vi "Get channel info.vi"(8 "error in":errorcluster) -> (0 "error out":errorcluster, 1 "Cancelled":bool, 3 "Sampling info":T1 {"Channels"."Hi cutoff" items=["500"=500.0, "1k"=1000.0, "5k"=5000.0, "10k"=10000.0, "20k"=20000.0]; "Channels"."Lo cutoff" items=["0.1"=0.1, "1"=1.0, "10"=10.0, "100"=100.0, "300"=300.0]; "Channels"."Gain" items=["x100"=100, "x1000"=1000, "x10000"=10000]})   [LabVIEW 2012]
uses:
  Channel.ctl
  Sampling info.ctl
panel:
  in  "Vel gain in":dbl=0.5 caption="Speed gain"
  in  "Pos gain in":dbl=1.0 caption="Position gain"
  in  "Max accel in":dbl[unit]=17453.292519943294 caption="Maximum acceleration"
  in  "Max speed in":dbl[unit]=87.26646259971648 caption="Maximum speed"
  in  "Steps bit in":u8 caption="Step bit"
  in  "Output frequency in":dbl[unit]=10000.0 caption="Output frequency"
  in  "Counts per rev in":i32=2048 caption="Encoder counts per revolution"
  in  "Motor driver in":string(combo)="US Digital MD2S" caption="Motor driver"
  in  "Steps per rev in":i32=6400 caption="Steps per revolution"
  in  "Cancel":bool
  in  "OK":bool
  in  "Amplifier in":string(combo)="A-M Systems 1700" caption="Amplifier"
  in  "Update frequency in":dbl[unit]=20.0 caption="Update frequency"
  in  "Sampling frequency in":dbl[unit]=5000.0 caption="Sampling frequency"
  in  "Channels in":T2[](array[typedef]) caption="Channels" {"Hi cutoff" items=["500"=500.0, "1k"=1000.0, "5k"=5000.0, "10k"=10000.0, "20k"=20000.0]; "Lo cutoff" items=["0.1"=0.1, "1"=1.0, "10"=10.0, "100"=100.0, "300"=300.0]; "Gain" items=["x100"=100, "x1000"=1000, "x10000"=10000]}
  # "Recording"
  # "Motor"
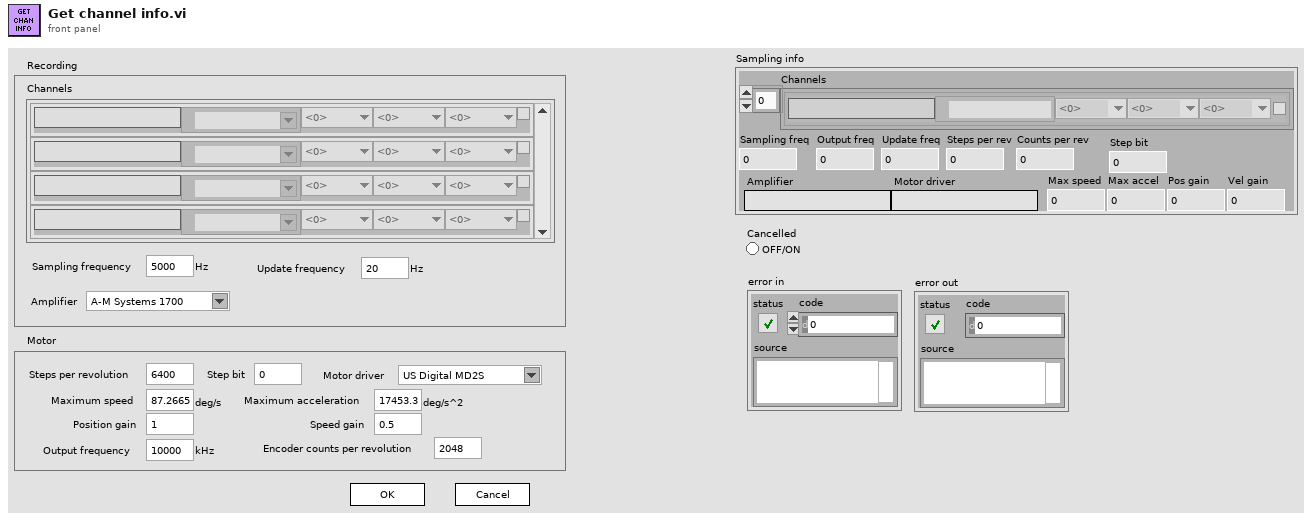
[diagram p1: front panel]
types:
  T1 = typedef "Sampling info.ctl" = cluster{"Channels":T2[], "Sampling freq":i32, "Output freq":i32, "Update freq":i32, "Steps per rev":i32, "Counts per rev":i32, "Amplifier":string, "Motor driver":string, "Step bit":u8, "Max speed":dbl, "Max accel":dbl, "Pos gain":dbl, "Vel gain":dbl}
  T2 = typedef "Channel.ctl" = cluster{"Name":string, "Chan":tag, "Gain":u16, "Lo cutoff":dbl, "Hi cutoff":dbl, "Notch":bool}
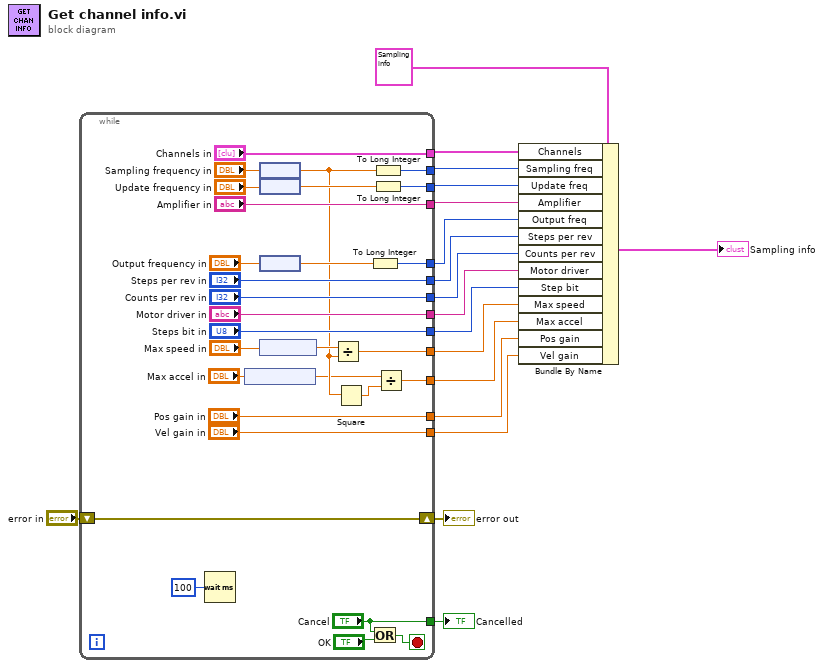
[diagram p0: block diagram]
diagram:
  n1 = while {
    tunnel: ["Cancel"] -> w8
    tunnel: ["Channels in"] -> w16
    tunnel: [w40] -> w17
    tunnel: [w39] -> w15
    tunnel: ["Amplifier in"] -> w14
    tunnel: [w34] -> w13
    tunnel: ["Steps per rev in"] -> w12
    tunnel: ["Counts per rev in"] -> w11
    tunnel: ["Motor driver in"] -> w10
    shift-right: [w30] -> w6
    shift-left: "error in" -> [w30]
    tunnel: ["Steps bit in"] -> w5
    tunnel: [w22] -> w4
    tunnel: [w21] -> w3
    tunnel: ["Pos gain in"] -> w2
    tunnel: ["Vel gain in"] -> w1
    stop <- w47 stop-if-true
    n2 = Wait (ms)(milliseconds to wait=u32 100) -> ()  [unwired: 1 out]
    n3 = node("Max accel in") -> (w23:dbl)
    n4 = node("Sampling frequency in") -> (w24:dbl)
    n5 = node("Update frequency in") -> (w37:dbl)
    n6 = node("Output frequency in") -> (w35:dbl)
    n7 = node("Max speed in") -> (w28:dbl)
    n8 = Divide(x=w28, y=w24) -> (x/y=w22:dbl)
    n9 = Square(x=w24) -> (x^2=w25:dbl)
    n10 = To Long Integer(number=w35) -> (32bit integer=w34:i32)
    n11 = Or(x="Cancel", y="OK") -> (x .or. y?=w47:bool)
    n12 = To Long Integer(number=w24) -> (32bit integer=w40:i32)
    n13 = To Long Integer(number=w37) -> (32bit integer=w39:i32)
    n14 = Divide(x=w23, y=w25) -> (x/y=w21:dbl)
  }
  "Cancelled" <- w8
  "error out" <- w6
  n15 = Bundle By Name(cluster=T1 {"Channels"=[], "Sampling freq"=0, "Output freq"=0, "Update freq"=0, "Steps per rev"=0, "Counts per rev"=0, "Amplifier"="", "Motor driver"="", "Step bit"=0, "Max speed"=0.0, "Max accel"=0.0, "Pos gain"=0.0, "Vel gain"=0.0} ("Sampling data"), "Channels"=w16, "Sampling freq"=w17, "Update freq"=w15, "Amplifier"=w14, "Output freq"=w13, "Steps per rev"=w12, "Counts per rev"=w11, "Motor driver"=w10, "Step bit"=w5, "Max speed"=w4, "Max accel"=w3, "Pos gain"=w2, "Vel gain"=w1) -> (→"Sampling info":T1)
